vi "Node - Initial Handshaking.vi"(8 "error in (no error)":errorcluster, 11 "Node Data In":T1) -> (0 "error out":errorcluster, 3 "Node Data Out":T1)   [LabVIEW 2016, in "PXImc Router.lvlib"]
uses:
  PXImc Router.lvlib
  Controls/Node Data.ctl
  Controls/Node/Node - PXImc Parameters.ctl
  Controls/Node/Node - Writer Data.ctl
  Controls/Node/Node Ch Properties.ctl
  Controls/Data Type.ctl
  Controls/Node/Node - Readers Data.ctl
  Controls/Node/Node - Reader Data.ctl
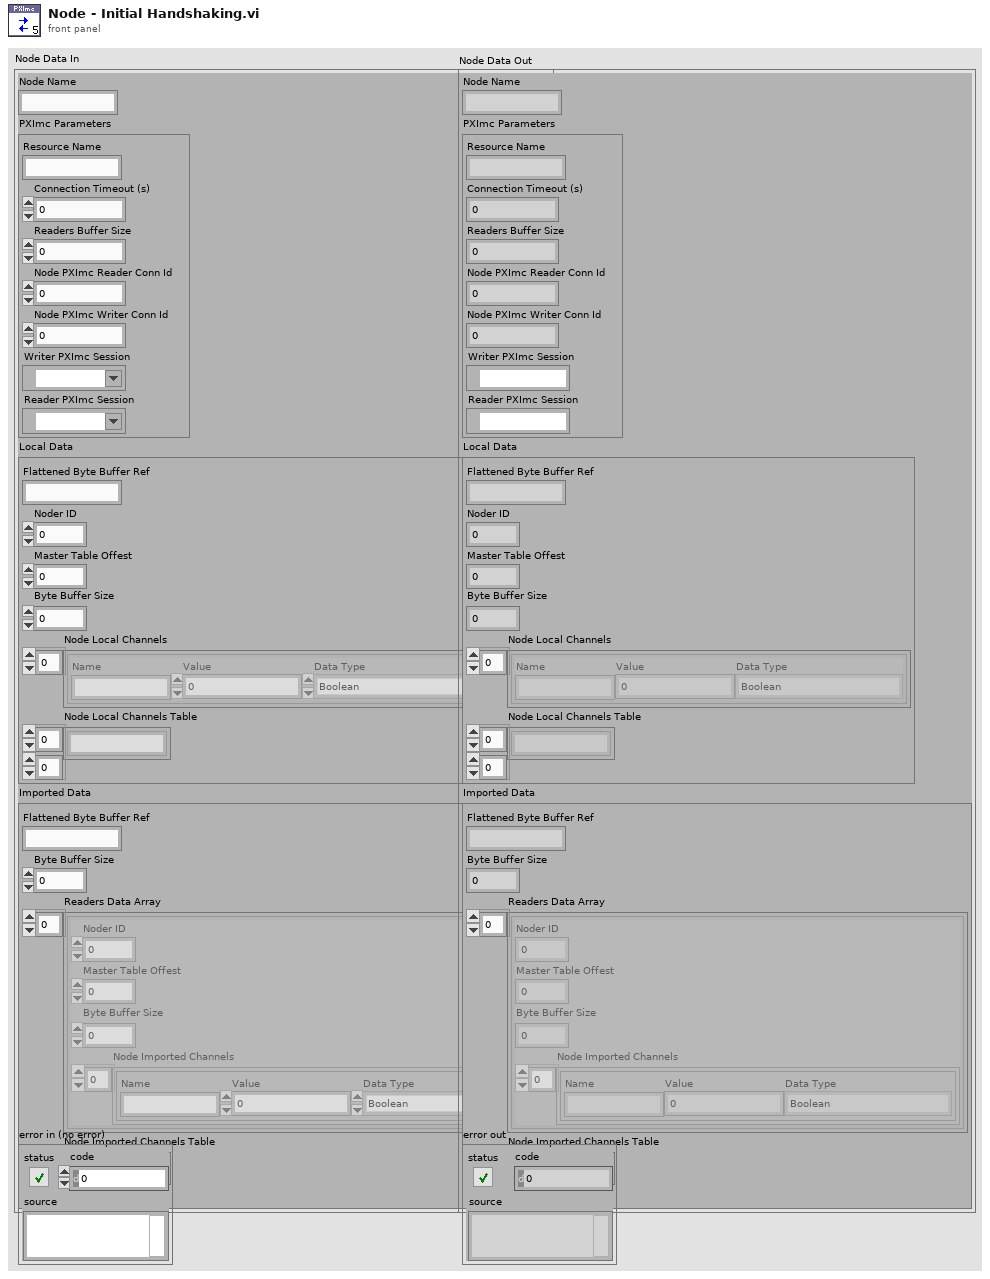
[diagram p1: front panel]
types:
  T1 = typedef "PXImc Router.lvlib/Node Data.ctl" = cluster{"Node Name":string, "PXImc Parameters":T2, "Local Data":T3, "Imported Data":T6}
  T2 = typedef "PXImc Router.lvlib/Node - PXImc Parameters.ctl" = cluster{"Resource Name":string, "Connection Timeout (s)":dbl, "Readers Buffer Size":u64, "Node PXImc Reader Conn Id":u16, "Node PXImc Writer Conn Id":u16, "Writer PXImc Session":refnum<k21>, "Reader PXImc Session":refnum<k21>}
  T3 = typedef "PXImc Router.lvlib/Node - Writer Data.ctl" = cluster{"Flattened Byte Buffer Ref":string, "Noder ID":u32, "Master Table Offest":u32, "Byte Buffer Size":u32, "Node Local Channels":T4[], "Node Local Channels Table":string[][]}
  T4 = typedef "PXImc Router.lvlib/Node Ch Properties.ctl" = cluster{"Name":string, "Value":dbl, "Data Type":T5}
  T5 = typedef "PXImc Router.lvlib/Data Type.ctl" = enum16{"Boolean", "SGL", "DBL", "I8", "I16", "I32", "I64", "U8", "U16", "U32", "U64"}
  T6 = typedef "PXImc Router.lvlib/Node - Readers Data.ctl" = cluster{"Flattened Byte Buffer Ref":string, "Byte Buffer Size":u64, "Readers Data Array":T7[], "Node Imported Channels Table":string[][]}
  T7 = typedef "PXImc Router.lvlib/Node - Reader Data.ctl" = cluster{"Noder ID":u32, "Master Table Offest":u32, "Byte Buffer Size":u64, "Node Imported Channels":T4[]}
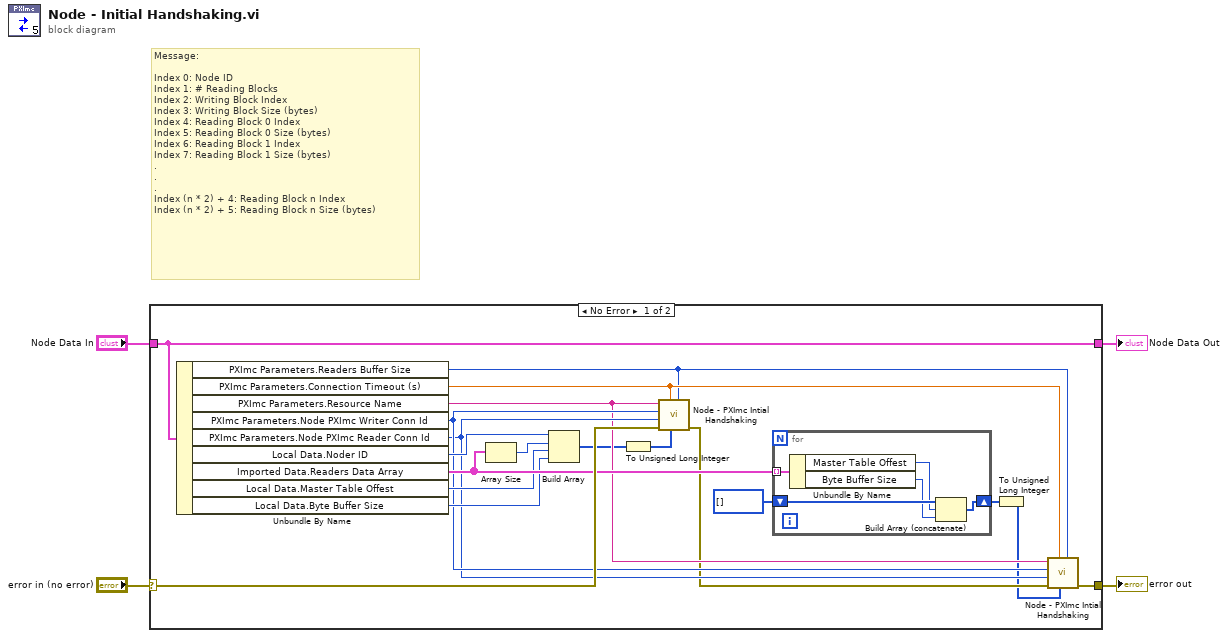
[diagram p0: block diagram]
diagram:
  # "Message:\n\nIndex 0: Node ID\nIndex 1: # Reading Blocks\nIndex 2: Writing Block Index\nIndex 3: Writing Block Size (bytes)\nIndex 4: Reading Block 0 Index\nIndex 5: Reading Block 0 Size (bytes)\nIndex 6: Reading Block 1 Index\nIndex 7: Reading Block 1 Size (bytes)\n.\n.\n.\nIndex (n * 2) + 4: Reading Block n Index\nIndex (n * 2) + 5: Reading Block n Size (bytes)"
  n1 = case shown="No Error" "error in (no error)" {
    selector: "error in (no error)" -> [w21 w30]
    tunnel: [w9 w30] -> w3
    tunnel: "Node Data In" -> [w23 w29]
    tunnel: [w23 w29] -> w1
    frame No Error {
      n2 = Unbundle By Name(w23) -> ("PXImc Parameters.Readers Buffer Size"=w14:u64, "PXImc Parameters.Connection Timeout (s)"=w15:dbl, "PXImc Parameters.Resource Name"=w11:string, "PXImc Parameters.Node PXImc Writer Conn Id"=w13:u16, "PXImc Parameters.Node PXImc Reader Conn Id"=w12:u16, "Local Data.Noder ID"=w20:u32, "Imported Data.Readers Data Array"=w19:T7[], "Local Data.Master Table Offest"=w17:u32, "Local Data.Byte Buffer Size"=w16:u32)
      n3 = Array Size(array=w19) -> (size(s)=w18:i32)
      n4 = Build Array(w20, w18, w17, w16) -> (w8:u32[])
      n5 = To Unsigned Long Integer(number=w8) -> (unsigned 32bit integer=w7:u32[])
      n6 = call "Node - PXImc Intial Handshaking.vi"("Reader Buffer Size In"=w14, "Data In"=w7, "Connection Timeout (s)"=w15, "error in (no error)"=w21, "Reader Conn ID"=w12, "Writer Conn ID"=w13, "Resource Name In"=w11) -> ("error out"=w10:errorcluster)  [unwired: 4 in]
      n7 = for {
        tunnel: w19 -> [w28] mode=indexing
        shift-right: [w24] -> w6
        shift-left: u32[] [] -> [w27]
        n8 = Unbundle By Name(w28) -> ("Master Table Offest"=w26:u32, "Byte Buffer Size"=w25:u64)
        n9 = Build Array (concatenate)(w27, w26, w25) -> (w24:u64[])
      }
      n10 = To Unsigned Long Integer(number=w6) -> (unsigned 32bit integer=w5:u32[])
      n11 = call "Node - PXImc Intial Handshaking.vi"("Reader Buffer Size In"=w14, "Data In"=w5, "Connection Timeout (s)"=w15, "error in (no error)"=w10, "Reader Conn ID"=w12, "Writer Conn ID"=w13, "Resource Name In"=w11) -> ("error out"=w9:errorcluster)  [unwired: 4 in]
    }
    frame Error {
    }
  }
  "Node Data Out" <- w1
  "error out" <- w3
